vi "Actor Core.vi"(8 "error in":errorcluster, 11 "Feeder":refnum<class "Feeder.lvclass">) -> (0 "error out":errorcluster, 3 "Actor out":refnum<class "Actor.lvclass">)   [LabVIEW 2018, in "Feeder Actor.lvlib" / "Feeder.lvclass"]
doc: "This is Actor Core.vi, the main message handling loop for Actors. An actor usually just sits in this loop and processes messages as they arrive. Any error returned by the message Do.vi call will stop the loop, with error code 43 as the canonical signal to stop with no error sent to caller. Descendants may override that in Handle Error.vi."
uses:
  Feeder.lvclass
  C:/Program Files/National Instruments/LabVIEW 2018/vi.lib/MGI/Panel Manager/Panel Actor/Panel Actor/Panel Actor.lvclass
  <vilib>/ActorFramework/Actor/Actor.lvclass
  Feeder.lvclass/Feeder.ctl
  <vilib>/MGI/Panel Manager/Panel Actor/Panel Actor/Panel Actor.lvclass
  ADM/Main.lvlib
  Mixer/Mixer.lvclass
  Screw/Screw.lvclass
  Solenoid/Solenoid.lvclass
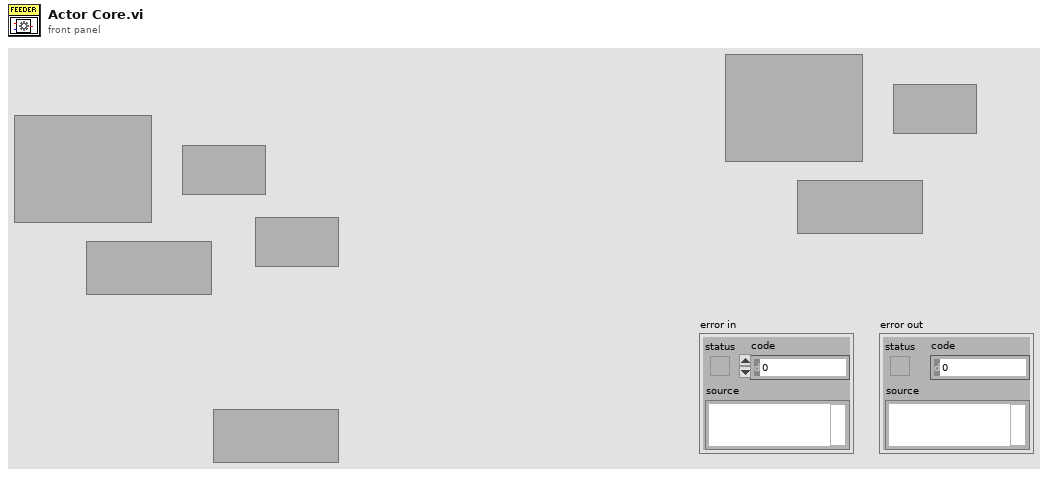
[diagram p1: front panel]
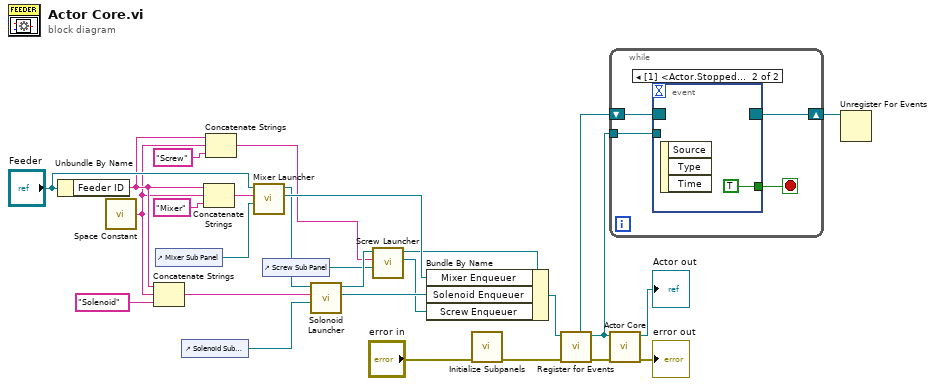
[diagram p0: block diagram]
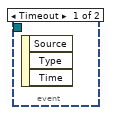
[diagram p2: hidden frame]
diagram:
  n1 = Unbundle By Name("Feeder") -> ("Feeder ID"=w8:string)
  n2 = call <vilib>:"Space Constant.vi"() -> ("String"=w7:string)
  n3 = Concatenate Strings(w8, w7, "Solenoid") -> (w2:string)
  n4 = control-ref of="Mixer Sub Panel"() -> (w14:refnum<vi>)
  n5 = control-ref of="Solenoid Sub Panel"() -> (w15:refnum<vi>)
  n6 = Concatenate Strings(w8, w7, "Mixer") -> (w1:string)
  n7 = Concatenate Strings(w8, w7, "Screw") -> (w3:string)
  n8 = call "Mixer Launcher.vi"("Sub Panel"=w14, "Mixer ID"=w1, "Feeder Actor In"="Feeder") -> ("Nested Actor's Enqueuer"=w19:refnum<class "Message Enqueuer.lvclass">, "Feeder Actor Out"=w16:refnum<class "Feeder.lvclass">)  [unwired: 7 in]
  n9 = control-ref of="Screw Sub Panel"() -> (w13:refnum<vi>)
  n10 = call "Solonoid Launcher.vi"("Sub Panel"=w15, "Solenoid ID"=w2, "Feeder Actor In"=w16) -> ("Nested Actor's Enqueuer"=w11:refnum<class "Message Enqueuer.lvclass">, "Feeder Actor Out"=w17:refnum<class "Feeder.lvclass">)  [unwired: 7 in]
  n11 = call "Screw Launcher.vi"("Sub Panel"=w13, "Screw ID"=w3, "Feeder Actor In"=w17) -> ("Nested Actor's Enqueuer"=w10:refnum<class "Message Enqueuer.lvclass">, "Feeder Actor Out"=w18:refnum<class "Feeder.lvclass">)  [unwired: 7 in]
  n12 = Bundle By Name(cluster=w18, "Mixer Enqueuer"=w19, "Solenoid Enqueuer"=w11, "Screw Enqueuer"=w10) -> (w12:refnum<class "Feeder.lvclass">)
  n13 = call "Initialize Subpanels.vi"("error in (no error)"="error in") -> ("error out"=w20:errorcluster)  [unwired: 10 in]
  n14 = call <vilib>:"Register for Events.vi"("Error In"=w20, "Panel Actor in"=w12) -> ("Error Out"=w23:errorcluster, "Panel Actor out"=w22:refnum<class "Feeder.lvclass">, "Pnl Actor"=w21:refnum<event-registration>)  [unwired: 6 in, 1 out]
  n15 = while {
    shift-right: [w29] -> w25
    shift-left: w21 -> [w31]
    tunnel: w22 -> [w28]
    stop <- w30 stop-if-true
    n16 = event shown="[1] <Actor.Stopped>: User Event" {
      selector: w31 -> [_ _]
      dyn-events: [_ _] -> w29
      timeout: _ -> [_ _]
      tunnel: [_ TRUE] -> w30
      tunnel: w28 -> [_ _]
      event Timeout {
        n17 = event-data() -> ()  [unwired: 1 in, 3 out]
      }
      event User Event {
        n18 = event-data() -> ()  [unwired: 1 in, 3 out]
      }
    }
  }
  n19 = call-parent "Actor Core.vi"("error in"=w23, "Panel Actor in"=w22) -> ("error out"=→"error out":errorcluster, "Actor out"=→"Actor out":refnum<class "Actor.lvclass">)  [unwired: 8 in]
  n20 = Unregister For Events(event registration refnum=w25) -> ()  [unwired: 1 in, 1 out]
